vi "Menu_In Place Bundler.vi"(11 "Affected Items Out":T1) -> (3 "Menu Items To Add":T2(array[cluster]))   [LabVIEW 2023]
uses:
  top/BundleMagic.ctl
  controls/action enum.ctl
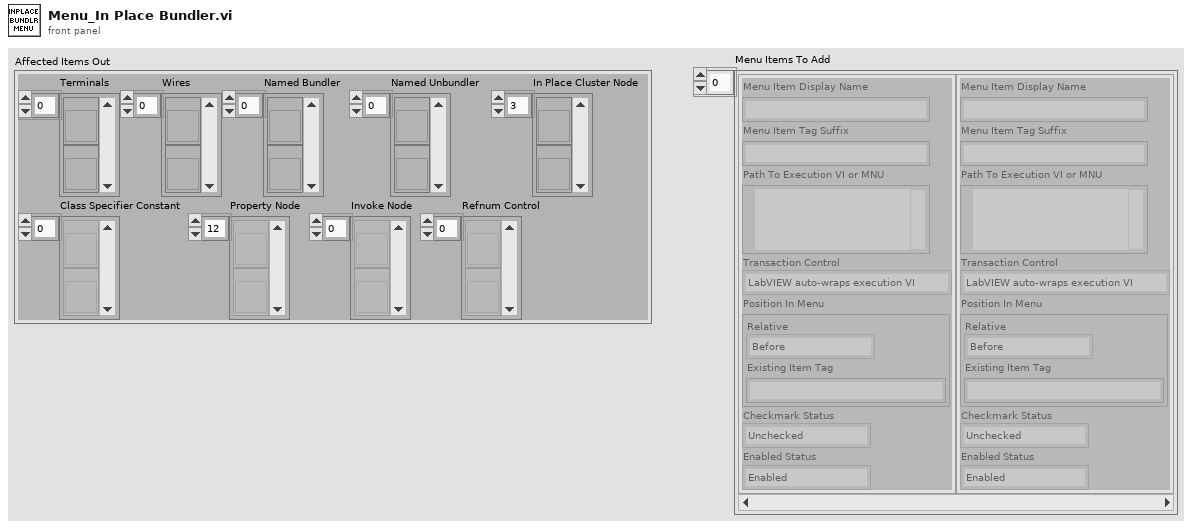
[diagram p1: front panel]
types:
  T1 = typedef "BundleMagic.ctl" = cluster{"Terminals":refnum<vi>[], "Wires":refnum<vi>[], "Named Bundler":refnum<vi>[], "Named Unbundler":refnum<vi>[], "In Place Cluster Node":refnum<vi>[], "Class Specifier Constant":refnum<vi>[], "Property Node":refnum<vi>[], "Invoke Node":refnum<vi>[], "Refnum Control":refnum<vi>[]}
  T2 = cluster{"Menu Item Display Name":string, "Menu Item Tag Suffix":string, "Path To Execution VI or MNU":path, "Transaction Control":enum8{"LabVIEW auto-wraps execution VI", "Execution VI will define if needed"}, "Position In Menu":cluster{"Relative":enum8{"Before", "Instead of", "After", "Into Submenu"}, "Existing Item Tag":string}, "Checkmark Status":enum8{"Unchecked", "Checked"}, "Enabled Status":enum8{"Enabled", "Disabled"}}[]
  T3 = typedef "action enum.ctl" = enum16{"[NONE]", "APP_SEPARATOR", "Wire Bundle", "Wire Unbundle", "Terminal Unbundle", "Terminal Bundle", "Bundler Move Up", "Bundler Move Down", "Bundler Insert", "Bundler Remove", "Bundler Remove Unwired", "Bundler Reorder", "In Place Insert", "In Place Remove", "In Place Remove Unwired", "In Place Reorder", "Wire Properties", "Wire Method", "Terminal Properties", "Terminal Method", "Property Move Up", "Property Move Down", "Properties Insert", "Properties Remove", "Properties Remove Unwired", "Properties Reorder", "Method Change", "Class For Constant", "Class For Control", "Class For Node", "Class Name to Clipboard"}
  T4 = cluster{"Relative":enum8{"Before", "Instead of", "After", "Into Submenu"}, "Existing Item Tag":string}[]
  T5 = cluster{"Menu Item Display Name":string, "Menu Item Tag Suffix":string, "Path To Execution VI or MNU":path, "Transaction Control":enum8{"LabVIEW auto-wraps execution VI", "Execution VI will define if needed"}, "Position In Menu":cluster{"Relative":enum8{"Before", "Instead of", "After", "Into Submenu"}, "Existing Item Tag":string}, "Checkmark Status":enum8{"Unchecked", "Checked"}, "Enabled Status":enum8{"Enabled", "Disabled"}}
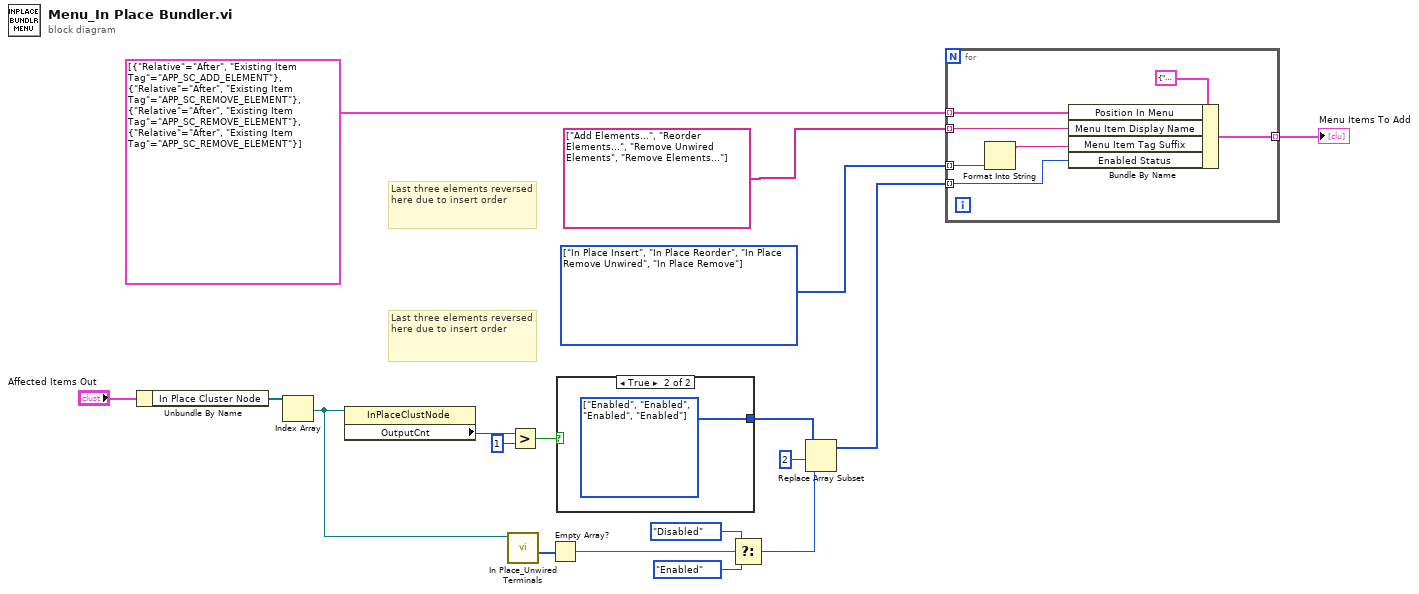
[diagram p0: block diagram]
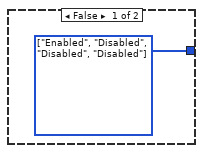
[diagram p2: hidden frame]
diagram:
  w1 = T3[] [enum."In Place Insert", enum."In Place Reorder", enum."In Place Remove Unwired", enum."In Place Remove"] items=["[NONE]", "APP_SEPARATOR", "Wire Bundle", "Wire Unbundle", "Terminal Unbundle", "Terminal Bundle", "Bundler Move Up", "Bundler Move Down", "Bundler Insert", "Bundler Remove", "Bundler Remove Unwired", "Bundler Reorder", "In Place Insert", "In Place Remove", "In Place Remove Unwired", "In Place Reorder", "Wire Properties", "Wire Method", "Terminal Properties", "Terminal Method", "Property Move Up", "Property Move Down", "Properties Insert", "Properties Remove", "Properties Remove Unwired", "Properties Reorder", "Method Change", "Class For Constant", "Class For Control", "Class For Node", "Class Name to Clipboard"] ("Enabled Status")
  # "Last three elements reversed here due to insert order"
  # "Last three elements reversed here due to insert order"
  n1 = Unbundle By Name("Affected Items Out") -> ("In Place Cluster Node"=w14:refnum<vi>[])
  n2 = Index Array(array=w14) -> (element=w4:refnum<vi>)  [unwired: 1 in]
  n3 = property class="InPlaceClustNode"(reference=w4) -> ("OutputCnt"=w12:i32)  [unwired: 1 in, 2 out]
  n4 = call "In Place_Unwired Terminals.vi"("In Place Node"=w4) -> ("Unwired Indices For Removal"=w3:u32[])  [unwired: 6 in, 4 out]
  n5 = Greater?(x=w12, y=1) -> (0:w9:bool)
  n6 = Empty Array?(array=w3) -> (empty?=w2:bool)
  n7 = case shown="True" w9 {
    tunnel: [w19 w20] -> w8
    frame False {
      w19 = enum8{"Enabled", "Disabled"}[] [enum."Enabled", enum."Disabled", enum."Disabled", enum."Disabled"] items=["Enabled", "Disabled"]
    }
    frame True {
      w20 = enum8{"Enabled", "Disabled"}[] [enum."Enabled", enum."Enabled", enum."Enabled", enum."Enabled"] items=["Enabled", "Disabled"]
    }
  }
  n8 = Select(t=enum8{"Enabled", "Disabled"}."Disabled" ("Enabled Status"), s=w2, f=enum8{"Enabled", "Disabled"}."Enabled" ("Enabled Status")) -> (s? t:f=w6:enum8{"Enabled", "Disabled"})
  n9 = Replace Array Subset(array=w8, new element=w6, index=2) -> (w7:enum8{"Enabled", "Disabled"}[])
  n10 = for {
    tunnel: [w27] -> w16 mode=indexing
    tunnel: string[] ["Add Elements...", "Reorder Elements...", "Remove Unwired Elements", "Remove Elements..."] -> [w26] mode=indexing
    tunnel: T4 [{"Relative"=enum."After", "Existing Item Tag"="APP_SC_ADD_ELEMENT"}, {"Relative"=enum."After", "Existing Item Tag"="APP_SC_REMOVE_ELEMENT"}, {"Relative"=enum."After", "Existing Item Tag"="APP_SC_REMOVE_ELEMENT"}, {"Relative"=enum."After", "Existing Item Tag"="APP_SC_REMOVE_ELEMENT"}] -> [w24] mode=indexing
    tunnel: w7 -> [w23] mode=indexing
    tunnel: w1 -> [w21] mode=indexing
    n11 = Format Into String(w21) -> (resulting string=w22:string)  [unwired: 3 in, 1 out]
    n12 = Bundle By Name(cluster=T5 {"Menu Item Display Name"="", "Menu Item Tag Suffix"="", "Path To Execution VI or MNU"=path "", "Transaction Control"=enum."LabVIEW auto-wraps execution VI", "Position In Menu"={"Relative"=enum."Before", "Existing Item Tag"=""}, "Checkmark Status"=enum."Unchecked", "Enabled Status"=enum."Enabled"} ("Cluster"), "Position In Menu"=w24, "Menu Item Display Name"=w26, "Menu Item Tag Suffix"=w22, "Enabled Status"=w23) -> (w27:T5)
  }
  "Menu Items To Add" <- w16
